vi "Set Use TSTRB.vi"(10 "value":bool, 11 "niInstr AXI4-Stream Reader v1 FPGA in":refnum<class "niInstr AXI4-Stream Reader v1 FPGA.lvclass">) -> (3 "niInstr AXI4-Stream Reader v1 FPGA out":refnum<class "niInstr AXI4-Stream Reader v1 FPGA.lvclass">)   [LabVIEW 2015, in "niInstr AXI4-Stream Reader v1 FPGA.lvclass"]
uses:
  <instrlib>/_niInstr/CLIP Adapters/v1/FPGA/AXI4-Stream/Reader/niInstr AXI4-Stream Reader v1 FPGA.lvclass
  <instrlib>/_niInstr/CLIP Adapters/v1/FPGA/AXI4-Stream/Reader/niInstr AXI4-Stream Reader v1 FPGA.lvclass/niInstr AXI4-Stream Reader v1 FPGA.ctl
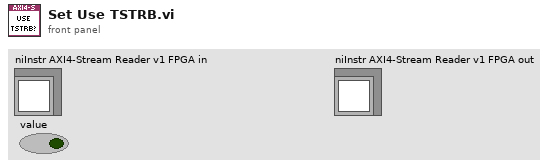
[diagram p1: front panel]
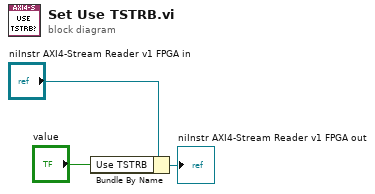
[diagram p0: block diagram]
diagram:
  n1 = Bundle By Name(cluster="niInstr AXI4-Stream Reader v1 FPGA in", "Use TSTRB"="value") -> (→"niInstr AXI4-Stream Reader v1 FPGA out":refnum<class "niInstr AXI4-Stream Reader v1 FPGA.lvclass">)
